vi "UseFGV1.vi"() -> ()   [LabVIEW 2019]
panel:
  in  "stop":bool
  out "Subscriber":dbl
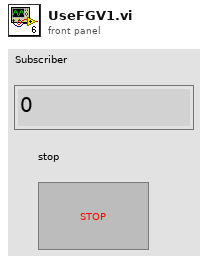
[diagram p1: front panel]
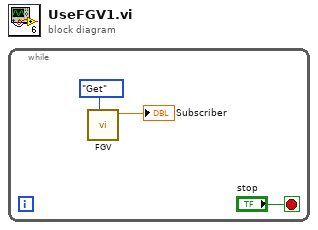
[diagram p0: block diagram]
diagram:
  n1 = while {
    stop <- "stop" stop-if-true
    n2 = call "FGV.vi"("State"=enum16{"Set", "Get"}."Get") -> ("Data Output"=→"Subscriber":dbl)  [unwired: 10 in]
  }
